vi "Read Event Ref.vi"(11 "Base Attributes in":refnum<class "Base Attributes.lvclass">) -> (2 "Event Ref":refnum<event-registration>)   [LabVIEW 2025, in "jettl.lvlib" / "Attributes.lvlib" / "Base Attributes.lvclass"]
uses:
  Base Attributes.lvclass
  Base Attributes.lvclass/Base Attributes.ctl
  Msg/Msg.lvclass
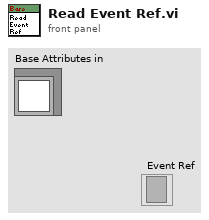
[diagram p1: front panel]
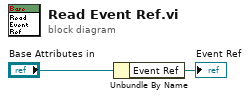
[diagram p0: block diagram]
diagram:
  n1 = Unbundle By Name("Base Attributes in") -> ("Event Ref"=→"Event Ref":refnum<event-registration>)
